vi "load single target.vi"(7 "database in":T5[](array[typedef]), 8 "error in":errorcluster, 11 "target to load":T1) -> (0 "error out":errorcluster, 3 "targets cluster out":T3)   [LabVIEW 2013, in "PLConfigurationSerializer.lvlib"]
uses:
  PLConfigurationSerializer.lvlib
  configuration database.ctl
  targets cluster.ctl
  target configuration/PL_Target Configuration.lvclass
  engines cluster.ctl
  <vilib>/NI/Module Execution Interface/Engine Configuration/engine configuration.lvclass
  <vilib>/NI/Tag Bus Module Framework/module configuration/TBM module configuration.lvclass
  target hierarchy.ctl
  engine hierarchy.ctl
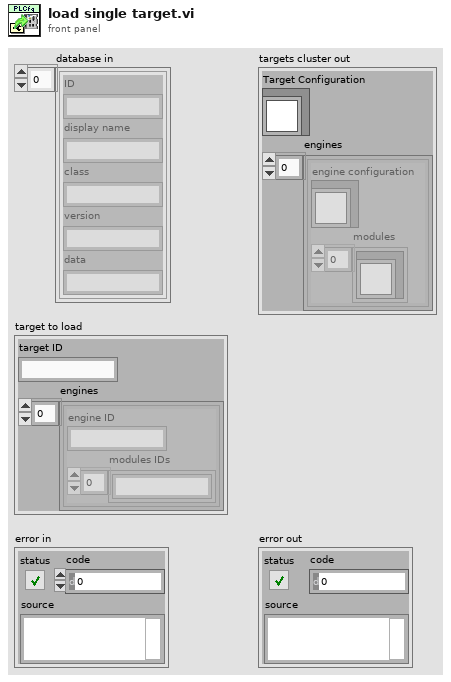
[diagram p1: front panel]
types:
  T1 = typedef "PLConfigurationSerializer.lvlib/target hierarchy.ctl" = cluster{"target ID":string, "engines":T2[]}
  T2 = typedef "PLConfigurationSerializer.lvlib/engine hierarchy.ctl" = cluster{"engine ID":string, "modules IDs":string[]}
  T3 = typedef "PLConfigurationSerializer.lvlib/targets cluster.ctl" = cluster{"Target Configuration":refnum<class "PL_Target Configuration.lvclass">, "engines":T4[]}
  T4 = typedef "PLConfigurationSerializer.lvlib/engines cluster.ctl" = cluster{"engine configuration":refnum<class "engine configuration.lvclass">, "modules":refnum<class "TBM module configuration.lvclass">[]}
  T5 = typedef "PLConfigurationSerializer.lvlib/configuration database.ctl" = cluster{"ID":string, "display name":string, "class":string, "version":string, "data":string}
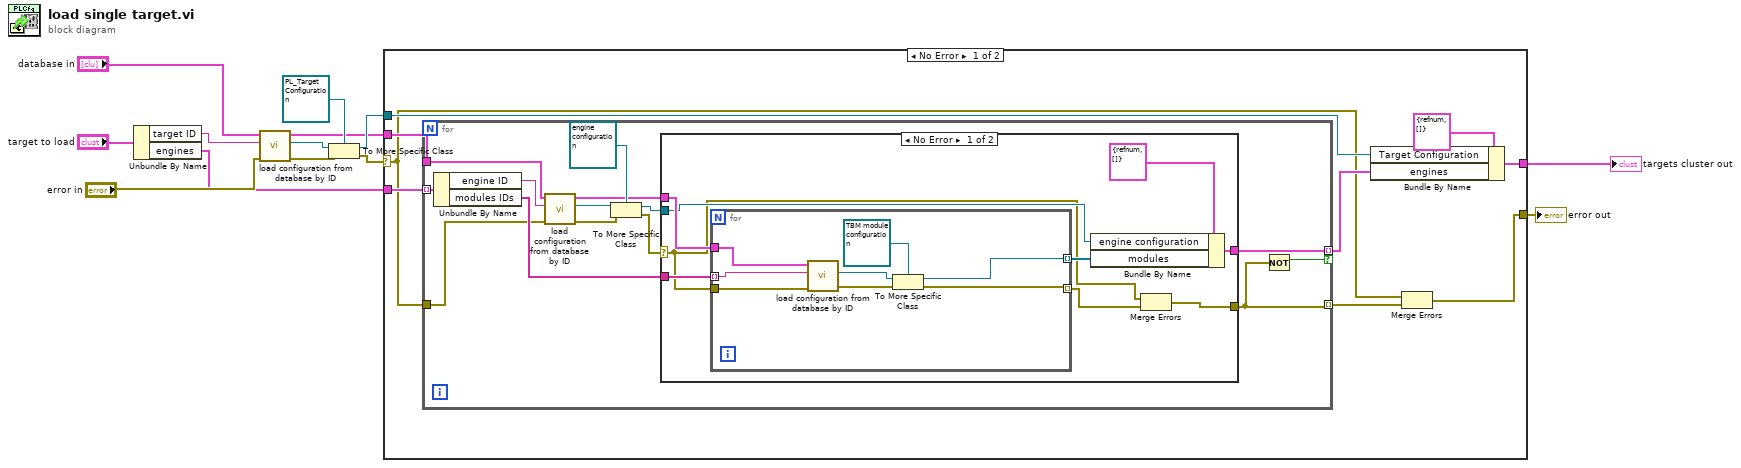
[diagram p0: block diagram]
diagram:
  n1 = Unbundle By Name("target to load") -> ("target ID"=w6:string, "engines"=w2:T2[])
  n2 = call "load configuration from database by ID.vi"("error in"="error in", "ID"=w6, "database in"="database in") -> ("error out"=w5:errorcluster, "configuration"=w4:refnum<class "TBM configuration.lvclass">, "database out"=w8:T5[])  [unwired: 6 in]
  n3 = To More Specific Class(target class=refnum<class "PL_Target Configuration.lvclass"> refnum ("Target Configuration"), reference=w4, error in=w5) -> (specific class reference=w13:refnum<class "PL_Target Configuration.lvclass">, error out=w10:errorcluster)
  n4 = case shown="No Error" w10 {
    selector: w10 -> [w14 w55]
    tunnel: w2 -> [w22 _]
    tunnel: [w19 _] -> w3
    tunnel: w8 -> [w18 _]
    tunnel: [w15 w55] -> w12
    tunnel: w13 -> [w17 _]
    frame No Error {
      n5 = for {
        tunnel: w22 -> [w36] mode=indexing
        tunnel: [w35] -> w20 mode=indexing if=w33
        tunnel: w18 -> [w29]
        tunnel: w14 -> [w26]
        tunnel: [w24] -> w16 mode=indexing
        n6 = Unbundle By Name(w36) -> ("engine ID"=w27:string, "modules IDs"=w34:string[])
        n7 = call "load configuration from database by ID.vi"("error in"=w26, "ID"=w27, "database in"=w29) -> ("error out"=w32:errorcluster, "configuration"=w31:refnum<class "TBM configuration.lvclass">, "database out"=w28:T5[])  [unwired: 6 in]
        n8 = To More Specific Class(target class=refnum<class "engine configuration.lvclass"> refnum ("engine configuration"), reference=w31, error in=w32) -> (specific class reference=w23:refnum<class "engine configuration.lvclass">, error out=w25:errorcluster)
        n9 = case shown="No Error" w25 {
          selector: w25 -> [w37 w54]
          tunnel: [w44 _] -> w35
          tunnel: w34 -> [w43 _]
          tunnel: w28 -> [w42 _]
          tunnel: [w38 w54] -> w24
          tunnel: w23 -> [w39 _]
          frame No Error {
            n10 = for {
              tunnel: w43 -> [w53] mode=indexing
              tunnel: w42 -> [w52]
              tunnel: [w47] -> w40 mode=indexing
              tunnel: w37 -> [w48]
              tunnel: [w49] -> w41 mode=indexing
              n11 = call "load configuration from database by ID.vi"("error in"=w48, "ID"=w53, "database in"=w52) -> ("error out"=w51:errorcluster, "configuration"=w50:refnum<class "TBM configuration.lvclass">)  [unwired: 6 in, 1 out]
              n12 = To More Specific Class(target class=refnum<class "TBM module configuration.lvclass"> refnum ("module configuration"), reference=w50, error in=w51) -> (specific class reference=w47:refnum<class "TBM module configuration.lvclass">, error out=w49:errorcluster)
            }
            n13 = Bundle By Name(cluster=T4 {"engine configuration"=refnum, "modules"=[]} ("engines cluster"), "engine configuration"=w39, "modules"=w40) -> (w44:T4)
            n14 = Merge Errors(w37, w41) -> (w38:errorcluster)
          }
          frame Error {
          }
        }
        n15 = Not(x=w24) -> (.not. x?=w33:bool)
      }
      n16 = Bundle By Name(cluster=T3 {"Target Configuration"=refnum, "engines"=[]} ("targets cluster"), "Target Configuration"=w17, "engines"=w20) -> (w19:T3)
      n17 = Merge Errors(w14, w16) -> (w15:errorcluster)
    }
    frame Error {
    }
  }
  "error out" <- w12
  "targets cluster out" <- w3
